vi "Update Chat Position.vi"(8 "error in (no error)":errorcluster, 10 "Message":variant, 11 "Telegram Class in":refnum<class "Telegram Class.lvclass">) -> (0 "error out":errorcluster, 3 "Telegram Class out":refnum<class "Telegram Class.lvclass">)   [LabVIEW 2015, in "Telegram Library.lvlib" / "Telegram Class.lvclass"]
doc: "Created IvanLis by LabVIEW Portal\nProfile: http://labviewportal.org/memberlist.php?mode=viewprofile&u=987\neMail: IvanLisanov@gMail.com\nTelegram: https://t.me/IvanLis"
uses:
  Telegram Class.lvclass
  JSON Library/TypeDef/ChatPosition.ctl
  TypeDef/Chat.ctl
  Telegram Class.lvclass/Telegram Class.ctl
  JSON Library/JSON Library.lvlib
  Telegram Library.lvlib
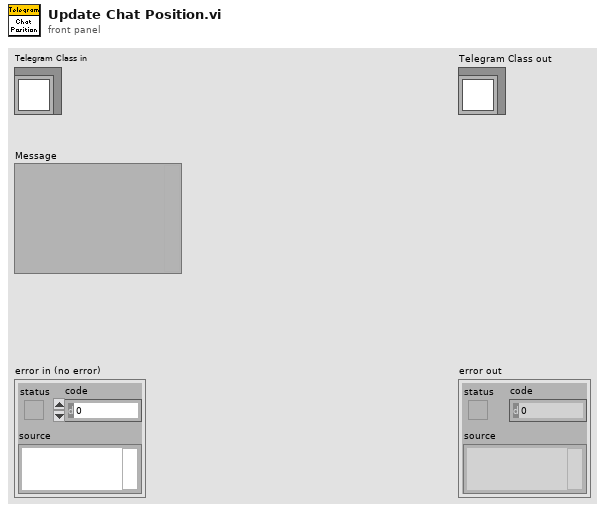
[diagram p1: front panel]
types:
  T1 = typedef "JSON Library.lvlib/ChatPosition.ctl" = cluster{"@type":string, "chat_id":i64, "position":cluster{"@type":string, "order":string}}
  T2 = typedef "Telegram Library.lvlib/Chat.ctl" = cluster{"id":i64, "position":i64, "title":string}
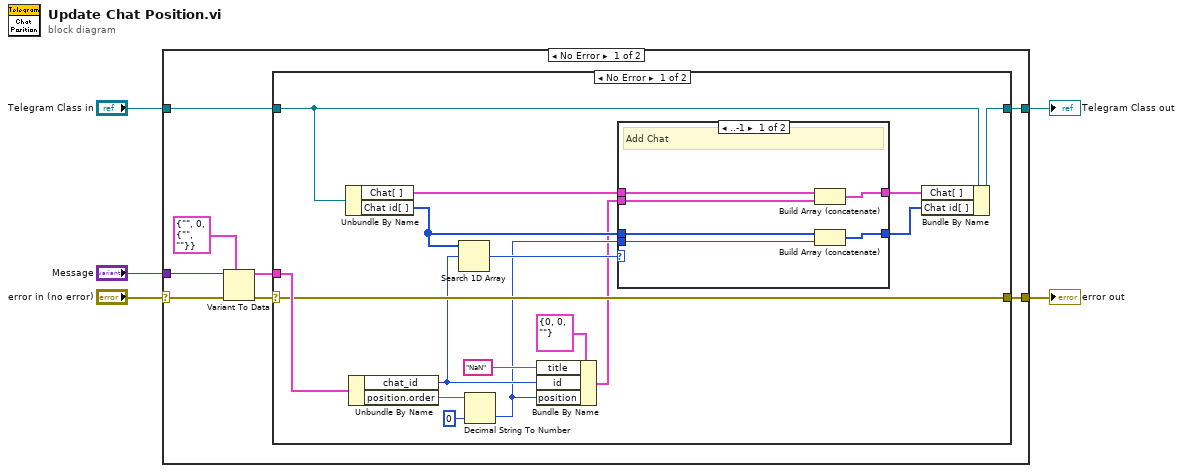
[diagram p0: block diagram]
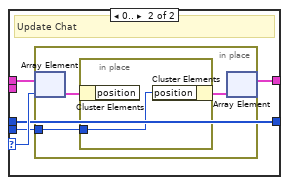
[diagram p2: hidden frame]
diagram:
  n1 = case shown="No Error" "error in (no error)" {
    selector: "error in (no error)" -> [w13 w48]
    tunnel: [w8 w48] -> w4
    tunnel: [w6 w47] -> w2
    tunnel: "Telegram Class in" -> [w7 w47]
    tunnel: "Message" -> [w11 _]
    frame No Error {
      n2 = Variant To Data(error in=w13, type=T1 {"@type"="", "chat_id"=0, "position"={"@type"="", "order"=""}} ("ChatPosition"), Variant=w11) -> (data=w10:T1, error out=w9:errorcluster)
      n3 = case shown="No Error" w9 {
        selector: w9 -> [w24 w46]
        tunnel: w10 -> [w29 _]
        tunnel: [w24 w46] -> w8
        tunnel: w7 -> [w28 w45]
        tunnel: [w18 w45] -> w6
        frame No Error {
          n4 = Unbundle By Name(w28) -> ("Chat[ ]"=w21:T2[], "Chat id[ ]"=w19:i64[])
          n5 = Unbundle By Name(w29) -> ("chat_id"=w23:i64, "position.order"=w26:string)
          n6 = Search 1D Array(1D array=w19, element=w23) -> (index of element=w22:i32)  [unwired: 1 in]
          n7 = Decimal String To Number(string=w26, default (0L)=i64 0 ("default (0 I32)")) -> (number=w20:i64)  [unwired: 1 in, 1 out]
          n8 = Bundle By Name(cluster=T2 {"id"=0, "position"=0, "title"=""} ("Chat"), "title"="NaN", "id"=w23, "position"=w20) -> (w15:T2)
          n9 = case shown="..-1" w22 {
            selector: w22 -> [_ w39]
            tunnel: w21 -> [w35 w40]
            tunnel: [w34 w38] -> w17
            tunnel: w20 -> [w32 w37]
            tunnel: w19 -> [w33 w36]
            tunnel: [w31 w36] -> w16
            tunnel: w15 -> [w30 _]
            frame ..-1 {
              # "Add Chat"
              n10 = Build Array (concatenate)(w35, w30) -> (w34:T2[])
              n11 = Build Array (concatenate)(w33, w32) -> (w31:i64[])
            }
            frame 0.. {
              # "Update Chat"
              n12 = in-place {
                in-place-border: w37 -> [w41]
                n13 = in-place-array #1(w40, w39) -> (w43:T2)
                n14 = in-place {
                  in-place-border: w41 -> [w44]
                  n15 = in-place-cluster #2(w43) -> ()  [unwired: 1 out]
                  n16 = in-place-cluster #2("position"=w44) -> (w42:T2)
                }
                n17 = in-place-array #1(w42) -> (w38:T2[])  [unwired: 1 out]
              }
            }
          }
          n18 = Bundle By Name(cluster=w28, "Chat[ ]"=w17, "Chat id[ ]"=w16) -> (w18:refnum<class "Telegram Class.lvclass">)
        }
        frame Error {
        }
      }
    }
    frame Error {
    }
  }
  "error out" <- w4
  "Telegram Class out" <- w2
